vi "CCC Start Server.vi"(8 "error in (no error)":errorcluster, 10 "port (54444)":u16=54444) -> (0 "error out":errorcluster)   [LabVIEW 2010]
doc: "Initializes the CCC server process, which runs asynchronously from the rest of the application."
uses:
  NI_CCC.lvlib
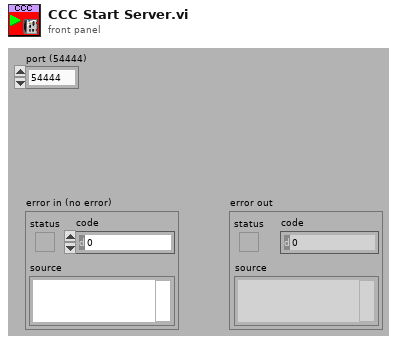
[diagram p1: front panel]
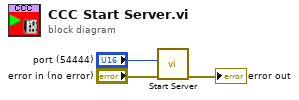
[diagram p0: block diagram]
diagram:
  n1 = call "Start Server.vi"("error in"="error in (no error)", "port (54444)"="port (54444)") -> ("error out"=→"error out":errorcluster)  [unwired: 9 in]
